vi "Master, Table Initialization.vi"(6 "Initialize (F)":bool, 7 "step name":string="Sequence Step General: Name", 8 "error in":errorcluster, 11 "Tbl Refnum":refnum<vi>) -> (0 "error out":errorcluster, 3 "Tbl Refnum dup":refnum<vi>)   [LabVIEW 2010]
panel:
  in  "Test Results":string[][](table) caption="Table 1"
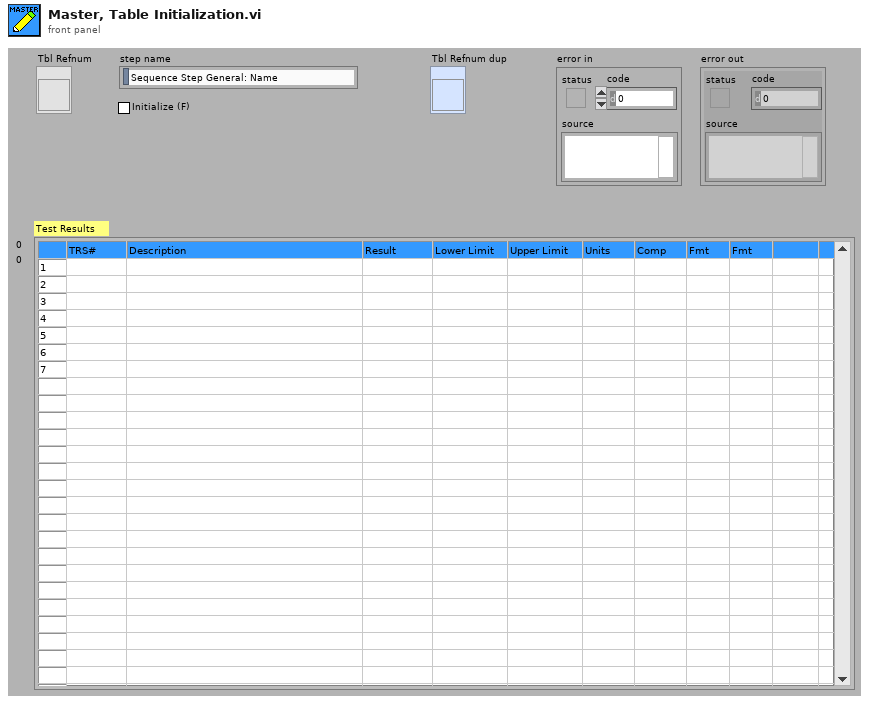
[diagram p1: front panel]
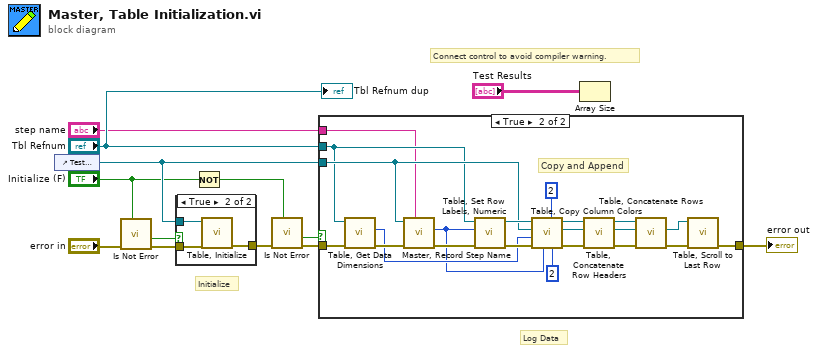
[diagram p0: block diagram]
diagram:
  # "Log Data"
  # "Initialize"
  # "Connect control to avoid compiler warning."
  n1 = control-ref of="Test Results"() -> (w11:refnum<vi>)
  n2 = call "Is Not Error.vi"("enable (T)"="Initialize (F)", "error in"="error in") -> ("error out"=w7:errorcluster, "ready"=w6:bool)  [unwired: 4 in, 1 out]
  n3 = case shown="True" w6 {
    tunnel: w7 -> [w14 w17]
    tunnel: [w14 w16] -> w5
    tunnel: w11 -> [_ w15]
    frame False {
    }
    frame True {
      n4 = call "Table, Initialize.vi"("error in"=w17, "Tbl Refnum"=w15) -> ("error out"=w16:errorcluster)  [unwired: 8 in, 1 out]
    }
  }
  n5 = Not(x="Initialize (F)") -> (.not. x?=w2:bool)
  n6 = call "Is Not Error.vi"("enable (T)"=w2, "error in"=w5) -> ("error out"=w4:errorcluster, "ready"=w3:bool)  [unwired: 4 in, 1 out]
  n7 = case shown="True" w3 {
    tunnel: w11 -> [_ w29]
    tunnel: "Tbl Refnum" -> [_ w22]
    tunnel: [w18 w38] -> w13
    tunnel: w4 -> [w18 w24]
    tunnel: "step name" -> [_ w19]
    frame False {
    }
    frame True {
      # "Copy and Append"
      n8 = call "Table, Get Data Dimensions.vi"("error in"=w24, "Tbl Refnum"=w22) -> ("error out"=w23:errorcluster, "row_n"=w21:i32)  [unwired: 6 in, 2 out]
      n9 = call "Master, Record Step Name.vi"("step name"=w19, "error in"=w23, "Tbl Refnum"=w29) -> ("error out"=w33:errorcluster, "row_n (I32)"=w20:i32)  [unwired: 6 in, 1 out]
      n10 = call "Table, Set Row Labels, Numeric.vi"("error in"=w33, "start (0)"=w20, "Tbl Refnum"=w22) -> ("error out"=w32:errorcluster, "Tbl Refnum out"=w30:refnum<vi>)  [unwired: 7 in]
      n11 = call "Table, Copy Column Colors.vi"("dst col (0)"=2 ("src col (0)"), "src col (0)"=2, "dst row (0)"=w20, "error in"=w32, "n rows (1)"=w21, "Tbl Refnum Dst"=w29, "Tbl Refnum Src"=w30) -> ("error out"=w31:errorcluster, "Tbl Refnum Dst out"=w27:refnum<vi>, "Tbl Refnum Src out"=w28:refnum<vi>)  [unwired: 2 in]
      n12 = call "Table, Concatenate Row Headers.vi"("error in"=w31, "Tbl Refnum Dst"=w27, "Tbl Refnum Src"=w28) -> ("error out"=w36:errorcluster, "Tbl Refnum Dst out"=w35:refnum<vi>, "Tbl Refnum Src out"=w34:refnum<vi>)  [unwired: 2 in]
      n13 = call "Table, Concatenate Rows.vi"("error in"=w36, "Tbl Refnum Dst"=w35, "Tbl Refnum Src"=w34) -> ("error out"=w39:errorcluster, "Tbl Refnum Dst out"=w37:refnum<vi>)  [unwired: 2 in, 1 out]
      n14 = call "Table, Scroll to Last Row.vi"("error in"=w39, "Tbl Refnum"=w37) -> ("error out"=w38:errorcluster)  [unwired: 7 in, 2 out]
    }
  }
  "error out" <- w13
  n15 = Array Size(array="Test Results") -> ()  [unwired: 1 out]
  "Tbl Refnum dup" <- "Tbl Refnum"
